vi "lock-in input sweep_1022D.vi"() -> ()   [LabVIEW 2022 SP3]
uses:
  <vilib>/Analysis/baseanly.llb/Mean (DBL).vi
  <vilib>/Utility/file.llb/Write Delimited Spreadsheet (DBL).vi
  <vilib>/Analysis/NI_AALBase.lvlib
panel:
  out "Temperature Status":i32(ring)=1 items=["TemperatureUnknown"=0, "Stable"=1, "Tracking"=2, "Near"=5, "Chasing"=6, "Filling"=7, "Standby"=10, "Disabled"=13, "ImpedanceNotFunction"=14, "TempFailure"=15]
  out "Field Status":i32(ring)=4 items=["MagnetUnknown"=0, "StablePersistent"=1, "WarmingSwitch"=2, "CoolingSwitch"=3, "StableDriven"=4, "Iterating"=5, "Charging"=6, "Discharging"=7, "CurrentError"=8, "MagnetFailure"=15]
  out "Field":dbl=-0.1023246817290783
  out "Temperature":dbl=2.045465922355652
  out "Measuring":bool
  in  "path2 (folder + filename)":string="H:\\My Drive\\Lab\\Opticool\\Measurement\\NLH\\T dependence\\TaI29_A1112_B116"
  in  "Series Resistance":string="20kOhm"
  in  "path1 (folder + filename)":string="H:\\My Drive\\Lab\\Opticool\\Measurement\\NLH\\T dependence\\TaI27_A1016_B1516"
  out "XY Graph 8":cluster{dbl[], dbl[]}(graph)={[0.1], [0.0]}
  out "XY Graph 7":cluster{dbl[], dbl[]}(graph)={[0.1], [0.0]}
  out "XY Graph 6":cluster{dbl[], dbl[]}(graph)
  out "XY Graph 5":cluster{dbl[], dbl[]}(graph)={[0.1], [0.0]}
  out "phase 2B":dbl
  in  "Phase 2B":u16(ring)=9 items=["X", "Y", "R", "Theta", "Frequency", "Noise", "Xh1", "Yh1", "Rh1", "Theta h1", "Xh2", "Yh2", "Rh2", "Theta h2"]
  out "phase 2A":dbl
  in  "Phase 2A":u16(ring)=3 items=["X", "Y", "R", "Theta", "Frequency", "Noise", "Xh1", "Yh1", "Rh1", "Theta h1", "Xh2", "Yh2", "Rh2", "Theta h2"]
  out "para2A Measurement":dbl
  in  "Clear Plot 2A":bool
  in  "Parameter 2A":u16(ring)=2 items=["X", "Y", "R", "Theta", "Frequency", "Noise", "Xh1", "Yh1", "Rh1", "Theta h1", "Xh2", "Yh2", "Rh2", "Theta h2"]
  out "para2B Measurement":dbl
  in  "Clear Plot 2B":bool
  in  "Parameter 2B":u16(ring)=8 items=["X", "Y", "R", "Theta", "Frequency", "Noise", "Xh1", "Yh1", "Rh1", "Theta h1", "Xh2", "Yh2", "Rh2", "Theta h2"]
  in  "Two Lock-in ?":bool=TRUE
  in  "B frequency 2":dbl=267.77 format="%#_13g"
  in  "2B Input Connection (0: Single-Ended)":u16(ring)=1 items=["Single-Ended Voltage", "Differential Voltage", "1 MOhm Current Gain", "100 MOhm Current Gain"]
  in  "2B harmonic 1":u8=2
  in  "2B harmonic 2":u8=3
  in  "2B reference Manual Phase":dbl=-59.75
  in  "auto phase 2B":bool=TRUE
  in  "2B Sample time (s)":dbl=0.001 min=0.001 max=100.0 step=0.001
  in  "2B Sensitivity":u16(ring)=27 items=["1 nV/fA", "2 nV/fA", "5 nV/fA", "10 nV/fA", "20 nV/fA", "50 nV/fA", "100 nV/fA", "200 nV/fA", "500 nV/fA", "1 uV/pA", "2 uV/pA", "5 uV/pA", "10 uV/pA", "20 uV/pA", "50 uV/pA", "100 uV/pA", "200 uV/pA", "500 uV/pA", "1 mV/nA", "2 mV/nA", "5 mV/nA", "10 mV/nA", "20 mV/nA", "50 mV/nA", "100 mV/nA", "200 mV/nA", "500 mV/nA", "1 V/uA"]
  in  "Enable Sync Filter 2B (open when f<200Hz)":bool
  in  "2B Time Constant":u8(ring)=9 items=["10 us", "30 us", "100 us", "300 us", "1 ms", "3 ms", "10 ms", "30 ms", "100 ms", "300 ms", "1 s", "3 s", "10 s", "30 s", "100 s", "300 s", "1 ks", "3 ks"]
  in  "2B Reference Source":u8(ring)=3 items=["External", "Internal", "Internal Sweep", "Channel-A"]
  in  "2B Low Pass Filter Slope":u8(ring)=2 items=["6 dB/oct", "12 dB/oct", "18 db/oct", "24 dB/oct"]
  in  "2A frequency":dbl=267.77 format="%#_13g"
  in  "2A Input Connection (0: Single-Ended)":u16(ring)=1 items=["Single-Ended Voltage", "Differential Voltage", "1 MOhm Current Gain", "100 MOhm Current Gain"]
  in  "2A harmonic":u8=2
  in  "2A harmonic":u8=3
  in  "2A reference Manual Phase":dbl=-59.75
  in  "auto phase 2A":bool=TRUE
  in  "2A Reference Source":u8(ring)=1 items=["External", "Internal", "Internal Sweep"]
  in  "2A Sample time (s)":dbl=0.001 min=0.001 max=100.0 step=0.001
  in  "2A Time Constant":u8(ring)=9 items=["10 us", "30 us", "100 us", "300 us", "1 ms", "3 ms", "10 ms", "30 ms", "100 ms", "300 ms", "1 s", "3 s", "10 s", "30 s", "100 s", "300 s", "1 ks", "3 ks"]
  in  "Enable Sync Filter 2A (open when f<200Hz)":bool
  in  "2A Sensitivity":u16(ring)=27 items=["1 nV/fA", "2 nV/fA", "5 nV/fA", "10 nV/fA", "20 nV/fA", "50 nV/fA", "100 nV/fA", "200 nV/fA", "500 nV/fA", "1 uV/pA", "2 uV/pA", "5 uV/pA", "10 uV/pA", "20 uV/pA", "50 uV/pA", "100 uV/pA", "200 uV/pA", "500 uV/pA", "1 mV/nA", "2 mV/nA", "5 mV/nA", "10 mV/nA", "20 mV/nA", "50 mV/nA", "100 mV/nA", "200 mV/nA", "500 mV/nA", "1 V/uA"]
  in  "2A Low Pass Filter Slope":u8(ring)=2 items=["6 dB/oct", "12 dB/oct", "18 db/oct", "24 dB/oct"]
  in  "LOCKIN2 address":refnum<visa-resource-name>="COM3"
  in  "Temperature \n& Field Function":bool
  in  "Field Approach":i32(ring) items=["Linear", "NoOvershoot", "Oscillate"]
  in  "F Rate (Oe/s)":dbl=100.0 format="%#_13g"
  in  "Set F (Oe)":dbl format="%#_13g"
  in  "Mode":i32(ring) items=["Persistent", "Driven"]
  in  "Temperature Approach":i32(ring)=1 items=["FastSettle", "NoOvershoot"]
  in  "T  Rate (K/min)":dbl=10.0
  in  "Set  T  (K)":dbl=2.0
  in  "WaitForField":bool=TRUE
  in  "WaitForTemperature":bool=TRUE
  in  "Delay":dbl=5.0
  in  "Remote":bool=TRUE
  in  "IP Address":string="169.254.170.239"
  in  "1A Low Pass Filter Slope":u8(ring)=2 items=["6 dB/oct", "12 dB/oct", "18 db/oct", "24 dB/oct"]
  in  "1B Low Pass Filter Slope":u8(ring)=2 items=["6 dB/oct", "12 dB/oct", "18 db/oct", "24 dB/oct"]
  in  "1B Reference Source":u8(ring)=3 items=["External", "Internal", "Internal Sweep", "Channel-A"]
  in  "1B Time Constant":u8(ring)=9 items=["10 us", "30 us", "100 us", "300 us", "1 ms", "3 ms", "10 ms", "30 ms", "100 ms", "300 ms", "1 s", "3 s", "10 s", "30 s", "100 s", "300 s", "1 ks", "3 ks"]
  in  "Enable Sync Filter 1B (open f<200Hz)":bool
  in  "1B Sensitivity":u16(ring)=27 items=["1 nV/fA", "2 nV/fA", "5 nV/fA", "10 nV/fA", "20 nV/fA", "50 nV/fA", "100 nV/fA", "200 nV/fA", "500 nV/fA", "1 uV/pA", "2 uV/pA", "5 uV/pA", "10 uV/pA", "20 uV/pA", "50 uV/pA", "100 uV/pA", "200 uV/pA", "500 uV/pA", "1 mV/nA", "2 mV/nA", "5 mV/nA", "10 mV/nA", "20 mV/nA", "50 mV/nA", "100 mV/nA", "200 mV/nA", "500 mV/nA", "1 V/uA"]
  in  "1A Sensitivity":u16(ring)=27 items=["1 nV/fA", "2 nV/fA", "5 nV/fA", "10 nV/fA", "20 nV/fA", "50 nV/fA", "100 nV/fA", "200 nV/fA", "500 nV/fA", "1 uV/pA", "2 uV/pA", "5 uV/pA", "10 uV/pA", "20 uV/pA", "50 uV/pA", "100 uV/pA", "200 uV/pA", "500 uV/pA", "1 mV/nA", "2 mV/nA", "5 mV/nA", "10 mV/nA", "20 mV/nA", "50 mV/nA", "100 mV/nA", "200 mV/nA", "500 mV/nA", "1 V/uA"]
  in  "Enable Sync Filter 1A (open f<200Hz)":bool
  in  "1A Time Constant":u8(ring)=9 items=["10 us", "30 us", "100 us", "300 us", "1 ms", "3 ms", "10 ms", "30 ms", "100 ms", "300 ms", "1 s", "3 s", "10 s", "30 s", "100 s", "300 s", "1 ks", "3 ks"]
  out "XY Graph 4":cluster{dbl[], dbl[]}(graph)={[0.1], [18.0]}
  in  "Phase 1B":u16(ring)=9 items=["X", "Y", "R", "Theta", "Frequency", "Noise", "Xh1", "Yh1", "Rh1", "Theta h1", "Xh2", "Yh2", "Rh2", "Theta h2"]
  in  "Parameter 1B":u16(ring)=8 items=["X", "Y", "R", "Theta", "Frequency", "Noise", "Xh1", "Yh1", "Rh1", "Theta h1", "Xh2", "Yh2", "Rh2", "Theta h2"]
  out "phase 1B":dbl=18.0
  in  "Clear Plot 1B":bool
  out "XY Graph 3":cluster{dbl[], dbl[]}(graph)={[0.1], [0.0]}
  out "para1B Measurement":dbl
  out "XY Graph 2":cluster{dbl[], dbl[]}(graph)={[0.1], [18.672111582001435]}
  in  "1B Sample time (s)":dbl=0.001 min=0.001 max=100.0 step=0.001
  in  "1A Sample time (s)":dbl=0.001 min=0.001 max=100.0 step=0.001
  in  "Phase 1A":u16(ring)=3 items=["X", "Y", "R", "Theta", "Frequency", "Noise", "Xh1", "Yh1", "Rh1", "Theta h1", "Xh2", "Yh2", "Rh2", "Theta h2"]
  in  "Parameter 1A":u16(ring)=2 items=["X", "Y", "R", "Theta", "Frequency", "Noise", "Xh1", "Yh1", "Rh1", "Theta h1", "Xh2", "Yh2", "Rh2", "Theta h2"]
  in  "stabilization(S)":dbl=0.5 format="%#_13g"
  in  "1B frequency":dbl=267.77 format="%#_13g"
  in  "1B Input Connection (0: Single-Ended)":u16(ring)=1 items=["Single-Ended Voltage", "Differential Voltage", "1 MOhm Current Gain", "100 MOhm Current Gain"]
  in  "1B harmonic 1":u8=2
  in  "B harmonic 2":u8=3
  in  "1B reference Manual Phase":dbl=-59.75
  in  "auto phase 1B":bool=TRUE
  in  "1A frequency":dbl=267.77 format="%#_13g"
  in  "1A Input Connection (0: Single-Ended)":u16(ring)=1 items=["Single-Ended Voltage", "Differential Voltage", "1 MOhm Current Gain", "100 MOhm Current Gain"]
  in  "1A harmonic 1":u8=2
  in  "1A harmonic 2":u8=3
  in  "1A reference Manual Phase":dbl=-59.75
  in  "auto phase 1A":bool=TRUE
  in  "1A Reference Source":u8(ring)=1 items=["External", "Internal", "Internal Sweep"]
  out "phase 1A":dbl=18.672111582001435
  out "loop run":i32=1
  in  "loop #":i32=1
  in  "Save data or not":bool=TRUE
  in  "Clear Plot 1A":bool
  out "XY Graph":cluster{dbl[], dbl[]}(graph)={[0.1], [2.9721208903815985]}
  out "para1A Measurement":dbl=2.9721208903815985
  out "Sine voltage":dbl=0.1 format="%#_13g"
  in  "GATE STEP(mv)":i32=20
  in  "Sine Low Value (0V)":dbl=0.1
  in  "Sine High Value (0.001-5V)":dbl=3.0
  in  "lockin waiting (s)":dbl=0.1 format="%#_13g"
  in  "LOCKIN1 address":refnum<visa-resource-name>="COM4"
  # "Mesurement 1"
  # "Lock-in 1 Setting"
  # "Channel 1A"
  # "Channel 1B"
  # "Lock-in 2 Setting"
  # "Channel 2A"
  # "Channel 2B"
  # "Mesurement 2"
  # "Mesurement 1"
  # "Sine Sweep Setting (Channel 1A)"
  # "Temprature and Field Setting"
  # "Mesurement 2"
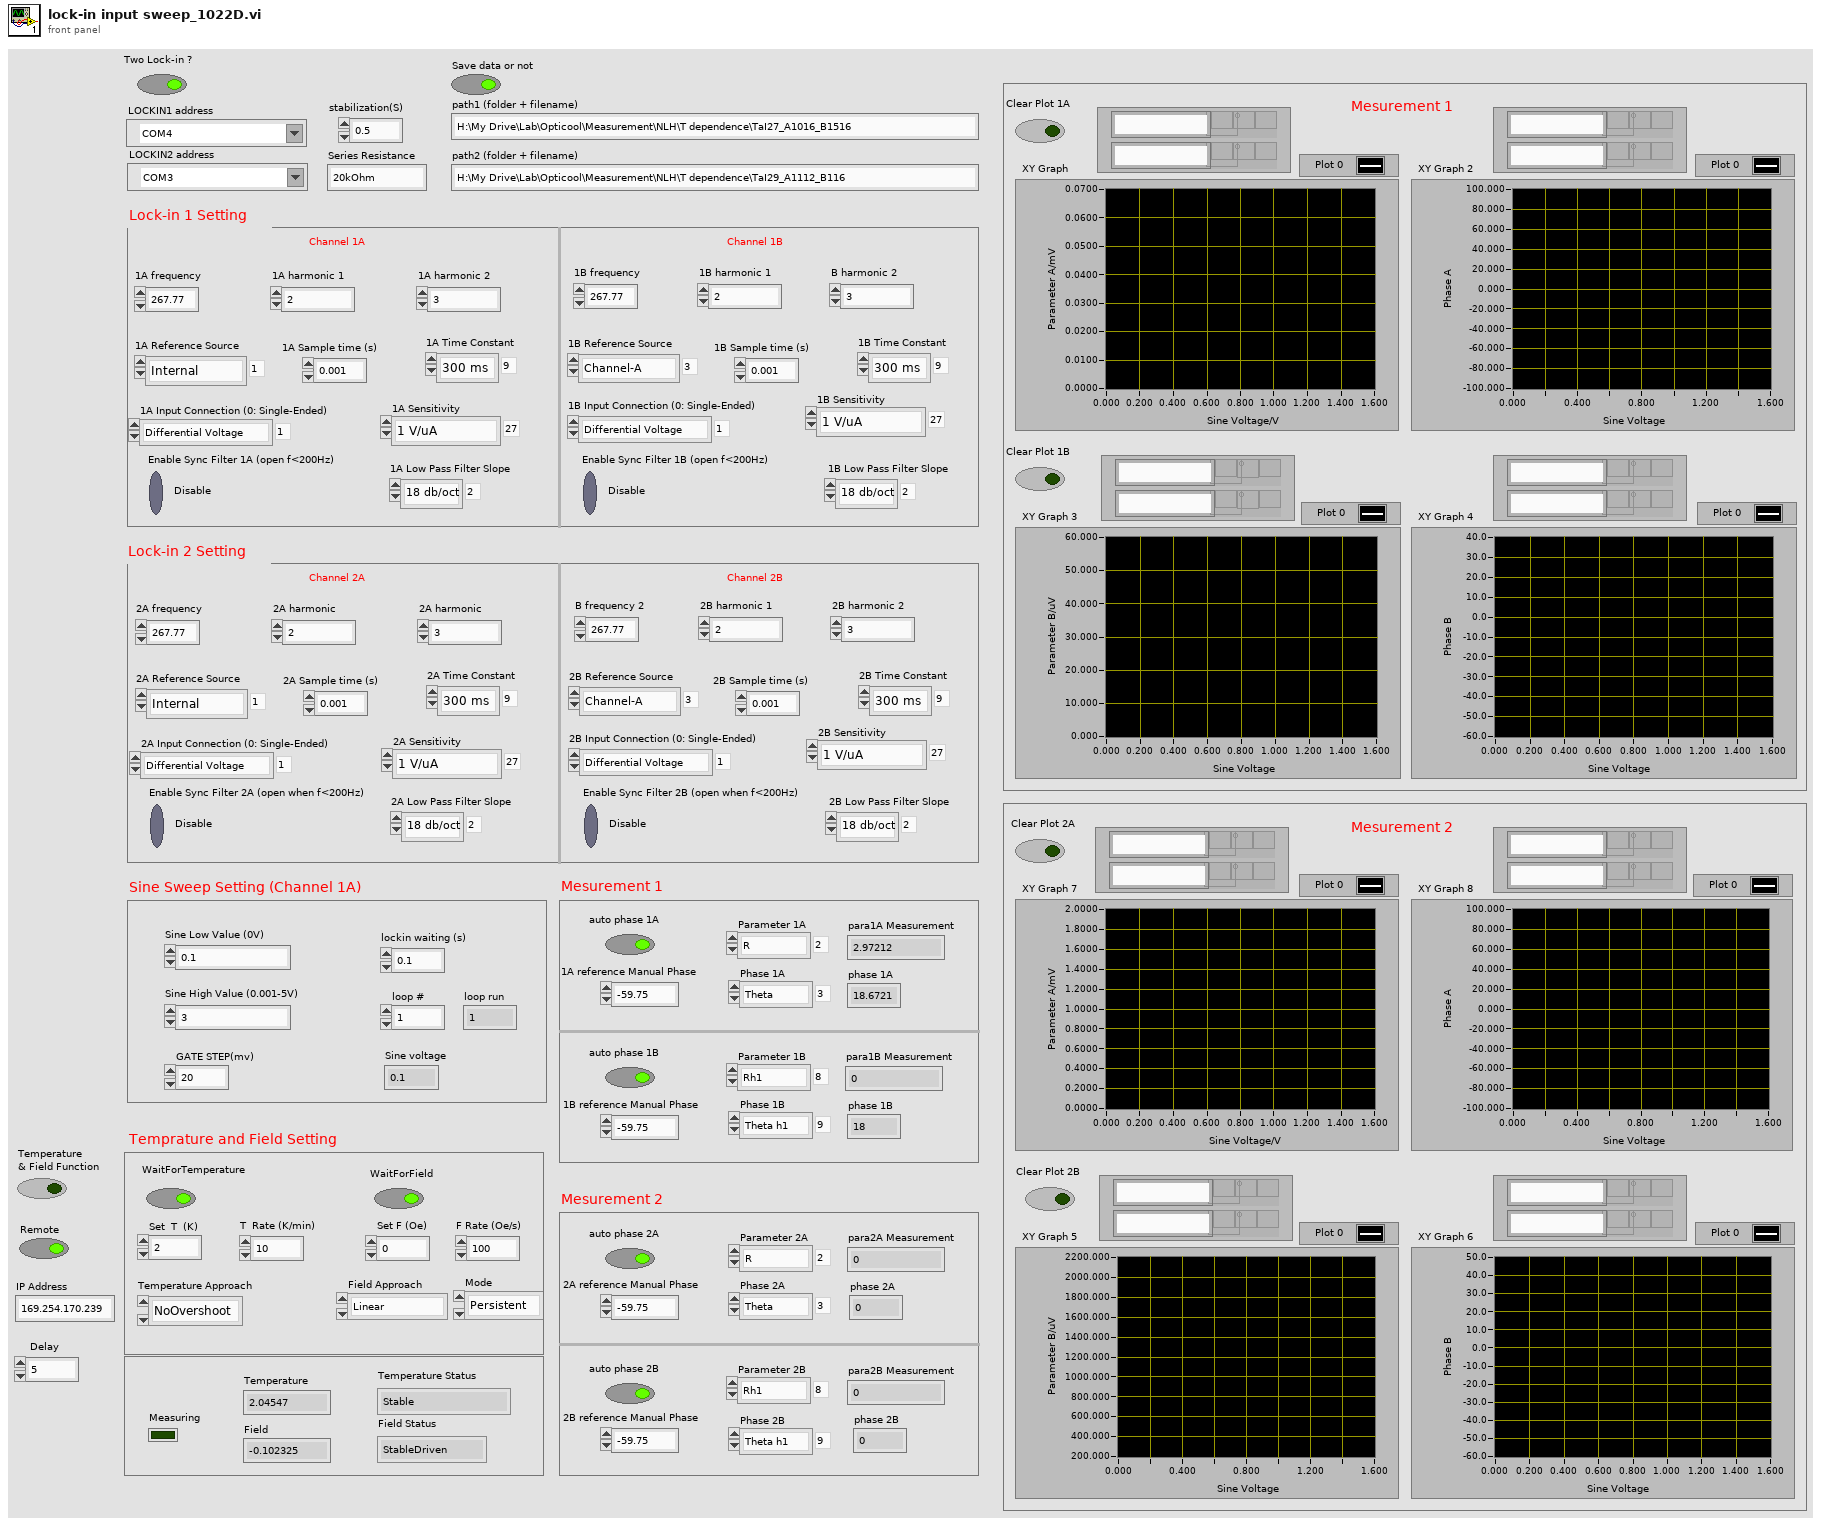
[diagram p1: front panel]
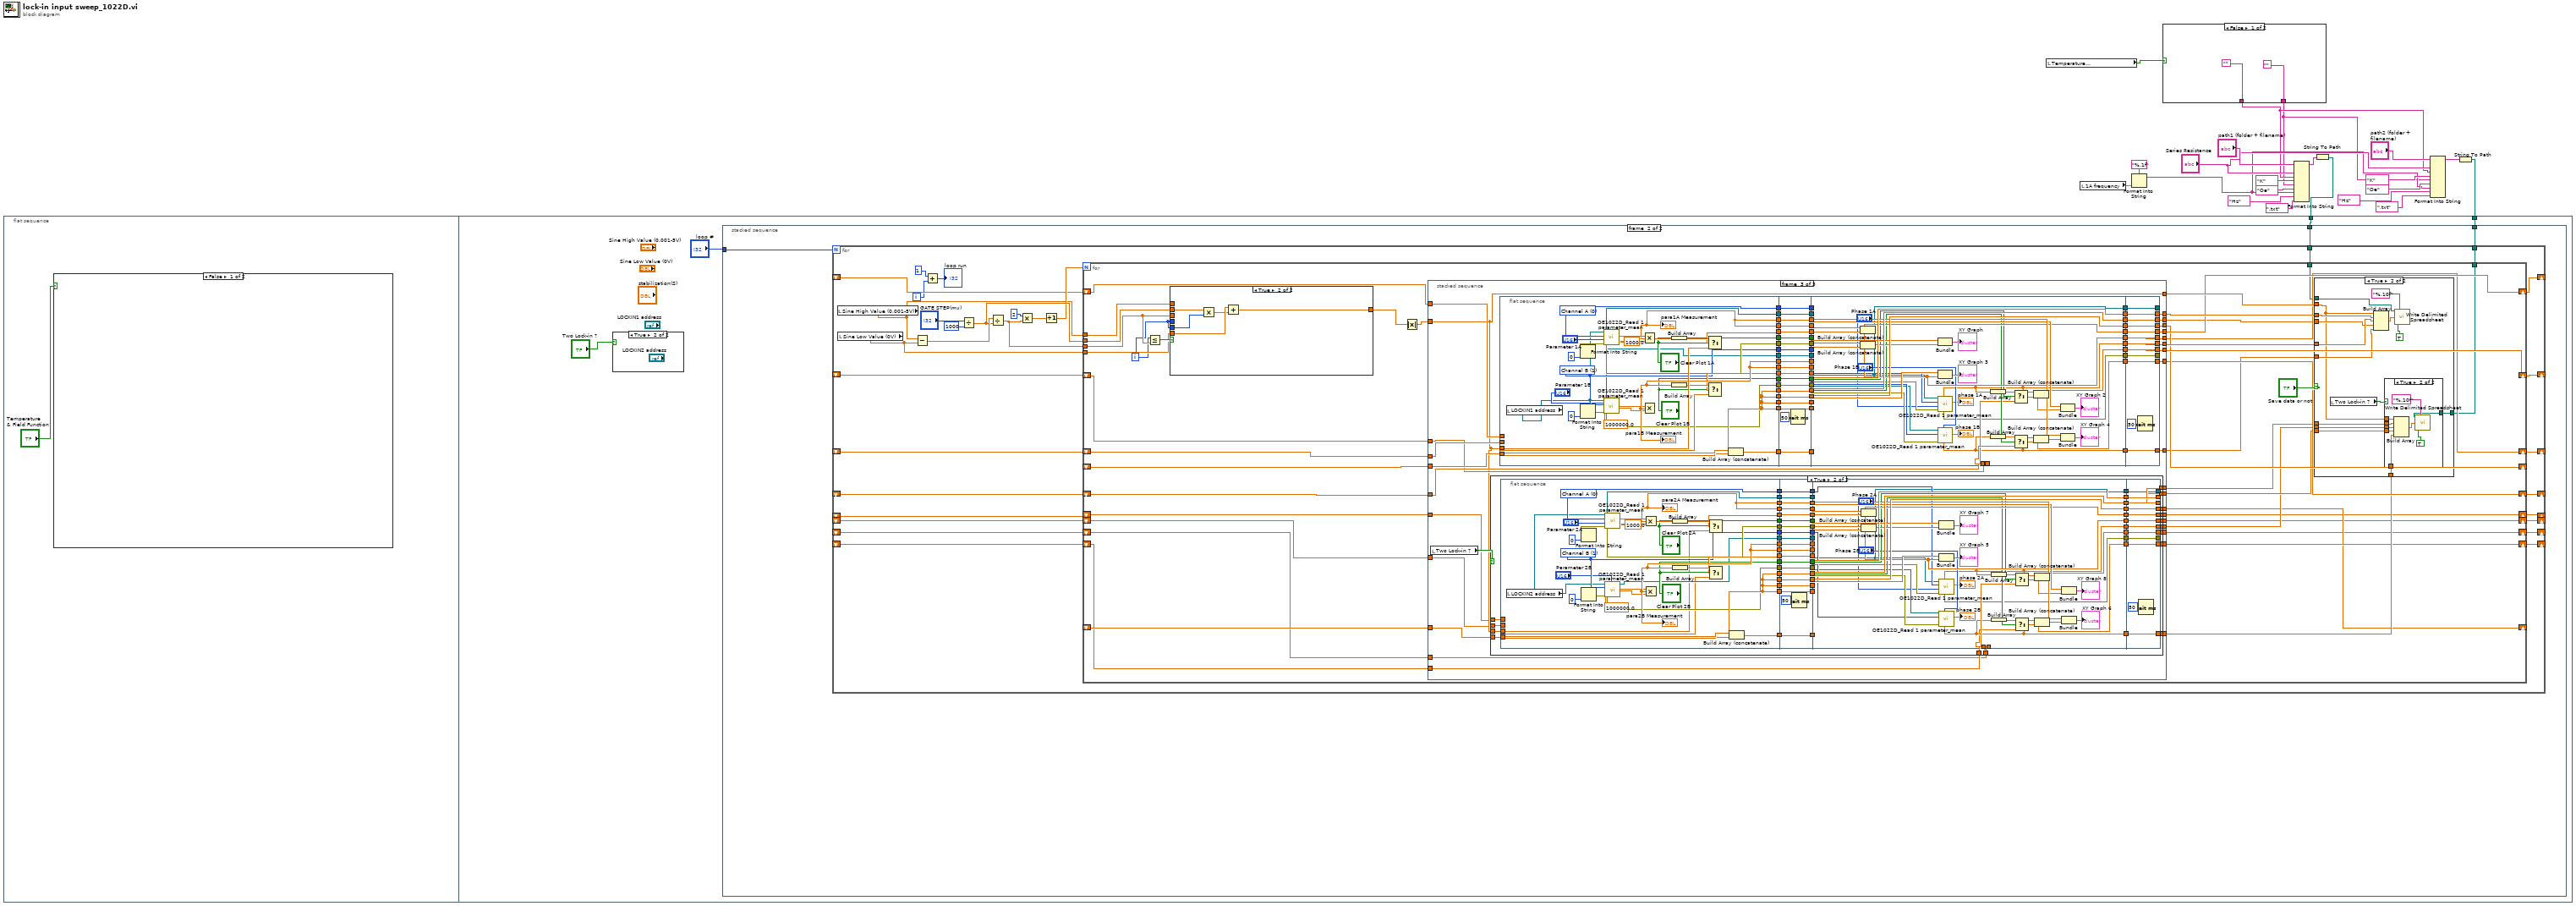
[diagram p0: block diagram]
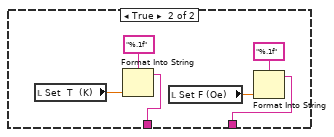
[diagram p2: hidden frame]
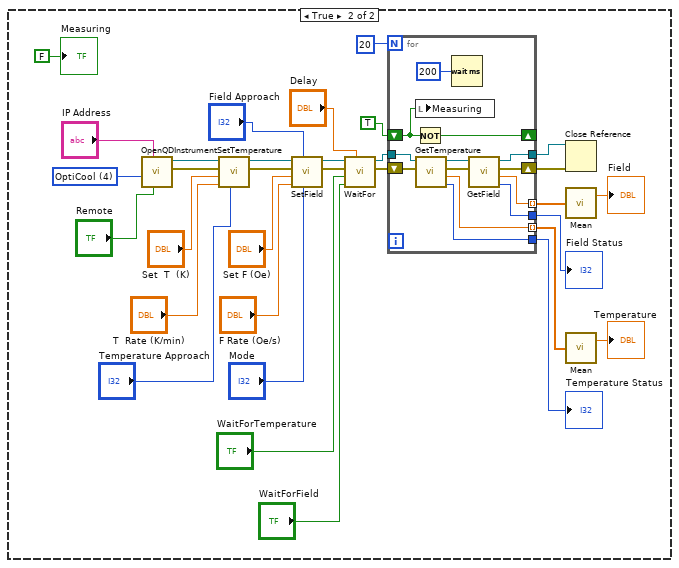
[diagram p3: hidden frame]
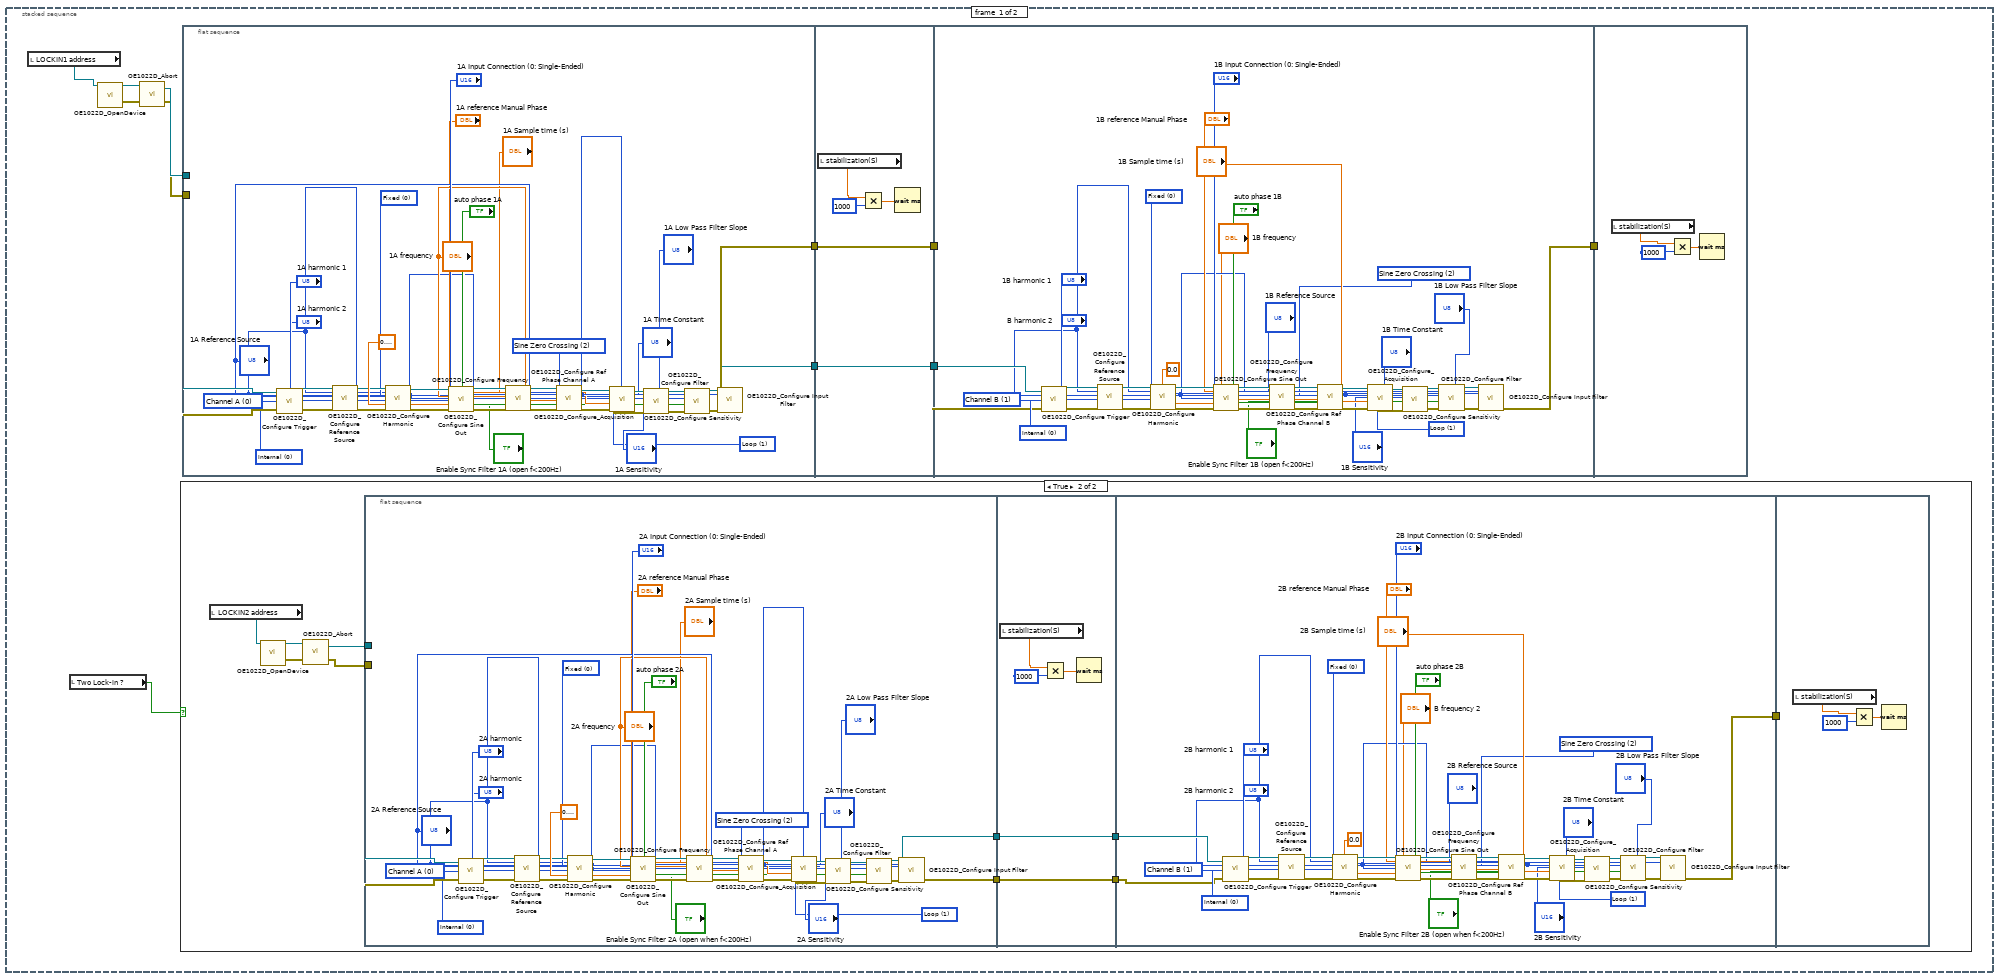
[diagram p5: hidden frame]
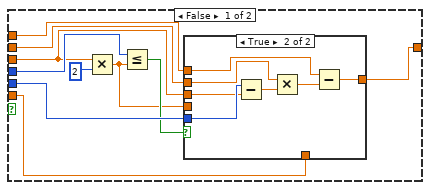
[diagram p9: hidden frame]
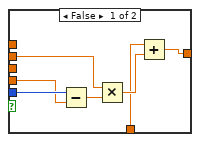
[diagram p10: hidden frame]
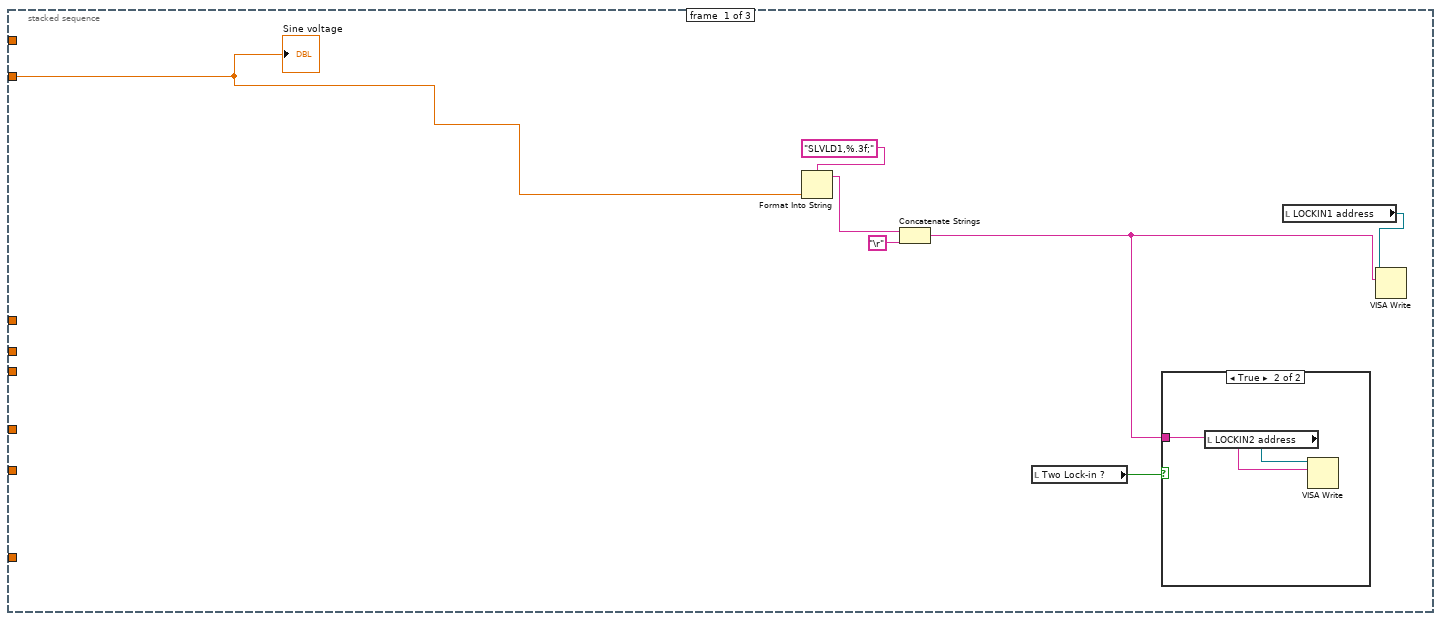
[diagram p11: hidden frame]
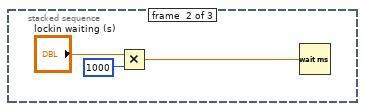
[diagram p13: hidden frame]
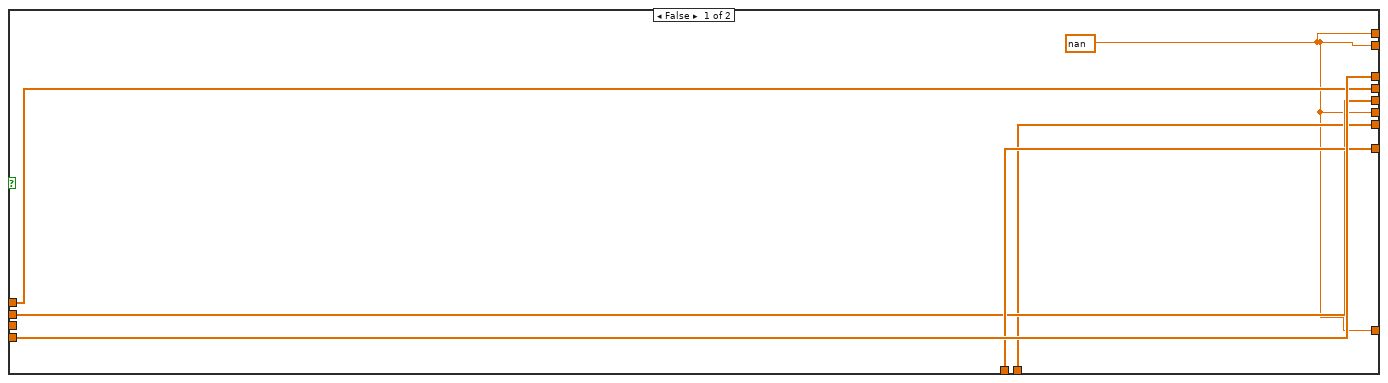
[diagram p14: hidden frame]
diagram:
  n1 = flat-sequence {
    tunnel: w16 -> [w69]
    tunnel: w1 -> [w68]
    frame #0 {
      n2 = case shown="False" "Temperature \n& Field Function" {
        frame False {
        }
        frame True {
          w46 = 4 items=["PPMS", "VersaLab", "DynaCool", "SVSM", "OptiCool"] ("InstrumentType")
          n3 = call "OpenQDInstrument.vi"("Remote"="Remote", "IP Address"="IP Address", "InstrumentType"=w46) -> ("error out"=w37:errorcluster, "Instrument Ref"=w38:refnum<k24>)  [unwired: 5 in]
          n4 = call "SetTemperature.vi"("Approach"="Temperature Approach", "Rate"="T  Rate (K/min)", "Temperature"="Set  T  (K)", "error in (no error)"=w37, "Instrument Ref In"=w38) -> ("error out"=w51:errorcluster, "Instrument Ref Out"=w50:refnum<k24>)  [unwired: 2 in, 1 out]
          n5 = call "SetField.vi"("Mode"="Mode", "Approach"="Field Approach", "Rate"="F Rate (Oe/s)", "Field"="Set F (Oe)", "error in (no error)"=w51, "Instrument Ref In"=w50) -> ("error out"=w33:errorcluster, "Instrument Ref Out"=w34:refnum<k24>)  [unwired: 1 in, 1 out]
          n6 = call "WaitFor.vi"("Delay"="Delay", "Wait For Field"="WaitForField", "Wait For Temperature"="WaitForTemperature", "error in (no error)"=w33, "Instrument Ref In"=w34) -> ("error out"=w45:errorcluster, "Instrument Ref Out"=w41:refnum<k24>)  [unwired: 5 in]
          n7 = for {
            N: 20 -> [_]
            shift-right: [w67] -> _
            shift-left: TRUE -> [w65]
            shift-right: [w62] -> w35
            shift-left: w45 -> [w64]
            tunnel: w41 -> [w61]
            tunnel: [w59] -> w36
            tunnel: [w56] -> w24
            tunnel: [w55] -> w23
            tunnel: [w57] -> w39 mode=indexing
            tunnel: [w58] -> w40 mode=indexing
            n8 = Not(x=w65) -> (.not. x?=w67:bool)
            n9 = local write "Measuring"(w65) -> ()
            n10 = call "GetTemperature.vi"("error in (no error)"=w64, "Instrument Ref In"=w61) -> ("Temperature\nStatus"=w55:i32, "Temperature"=w58:dbl, "error out"=w63:errorcluster, "Instrument Ref Out"=w60:refnum<k24>)  [unwired: 3 in, 1 out]
            n11 = Wait (ms)(milliseconds to wait=u32 200) -> ()  [unwired: 1 out]
            n12 = call "GetField.vi"("error in (no error)"=w63, "Instrument Ref In"=w60) -> ("Field\nStatus"=w56:i32, "Field"=w57:dbl, "error out"=w62:errorcluster, "Instrument Ref Out"=w59:refnum<k24>)  [unwired: 3 in, 1 out]
          }
          "Field Status" <- w24
          "Temperature Status" <- w23
          n13 = Close Reference(reference=w36, error in (no error)=w35) -> ()  [unwired: 1 out]
          n14 = call-poly <vilib>:"Mean.vi"("X"=w39) -> ("mean"=→"Field":dbl)  [unwired: 1 out]
          n15 = call-poly <vilib>:"Mean.vi"("X"=w40) -> ("mean"=→"Temperature":dbl)  [unwired: 1 out]
          "Measuring" <- FALSE
        }
      }
    }
    frame #1 {
      n16 = case shown="True" "Two Lock-in ?" {
        frame False {
        }
        frame True {
        }
      }
      n17 = stacked-sequence {
        tunnel: "loop #" -> [_ w269]
        tunnel: w69 -> [_ w268]
        tunnel: w68 -> [_ w267]
        frame #0 {
          n18 = local read "LOCKIN1 address"() -> (w73:refnum<visa-resource-name>)
          n19 = local read "Two Lock-in ?"() -> (w72:bool)
          n20 = call "OE1022D_OpenDevice.vi"("VISA resource name"=w73) -> ("VISA资源名称输出"=w74:refnum<visa-resource-name>, "错误输出"=w75:errorcluster)  [unwired: 17 in]
          n21 = call "OE1022D_Abort.vi"("error in (no error)"=w75, "VISA resource name"=w74) -> ("error out"=w80:errorcluster, "VISA resource name out"=w81:refnum<visa-resource-name>)
          n22 = case shown="True" w72 {
            frame False {
            }
            frame True {
              n23 = local read "LOCKIN2 address"() -> (w83:refnum<visa-resource-name>)
              n24 = call "OE1022D_OpenDevice.vi"("VISA resource name"=w83) -> ("VISA资源名称输出"=w86:refnum<visa-resource-name>, "错误输出"=w87:errorcluster)  [unwired: 17 in]
              n25 = call "OE1022D_Abort.vi"("error in (no error)"=w87, "VISA resource name"=w86) -> ("error out"=w84:errorcluster, "VISA resource name out"=w85:refnum<visa-resource-name>)
              n26 = flat-sequence {
                tunnel: w85 -> [w132]
                tunnel: [w120] -> w92
                tunnel: w84 -> [w131]
                tunnel: [w108] -> w91
                tunnel: w92 -> [w137]
                tunnel: [w137] -> w90
                tunnel: w91 -> [w136]
                tunnel: [w136] -> w89
                tunnel: w90 -> [w159]
                tunnel: [w158] -> w88
                tunnel: w89 -> [w157]
                tunnel: w88 -> [_]
                frame #0 {
                  w93 = u8 2 items=["TTL Pos", "TTL Neg", "Sine Zero Crossing"] ("External Ref Trigger")
                  w94 = u8 1 items=["Single", "Loop"] ("Sample Mode (Single/Loop)")
                  w107 = u8 0 items=["Fixed", "Linear", "Log"] ("SineOut Mode")
                  w109 = u16 0 items=["Internal", "External"] ("Trigger Source (0: Internal)")
                  w98 = u8 0 items=["Channel A", "Channel B"] ("OE1022D A/B")
                  n27 = call "OE1022D_Configure Trigger.vi"("Trigger Source (0: Internal)"=w109, "error in (no error)   2"=w131, "OE1022D A/B"=w98, "VISA resource name   2"=w132) -> ("error out   2"=w125:errorcluster, "VISA resource name out   2"=w126:refnum<visa-resource-name>)
                  n28 = call "OE1022D_Configure Reference Source.vi"("VISA resource name"=w126, "OE1022D A/B"=w98, "Reference Source"="2A Reference Source", "error in (no error)"=w125) -> ("VISA resource name out"=w124:refnum<visa-resource-name>, "error out"=w122:errorcluster)  [unwired: 14 in]
                  n29 = call "OE1022D_Configure Harmonic.vi"("VISA resource name"=w124, "OE1022D A/B"=w98, "Harmonic 1"="2A harmonic", "Harmonic 2"="2A harmonic", "error in (no error)"=w122) -> ("VISA resource name out"=w123:refnum<visa-resource-name>, "error out"=w121:errorcluster)  [unwired: 13 in]
                  n30 = call "OE1022D_Configure Sine Out.vi"("VISA resource name"=w123, "SineOut Mode"=w107, "OE1022D A/B"=w98, "Sine Output Amplitude (V)"=sgl 0.1, "error in (no error)"=w121) -> ("VISA resource name out"=w129:refnum<visa-resource-name>, "error out"=w128:errorcluster)  [unwired: 9 in]
                  n31 = call "OE1022D_Configure Frequency.vi"("VISA resource name"=w129, "OE1022D A/B"=w98, "Internal Frequency(Hz)"="2A frequency", "error in (no error)"=w128) -> ("VISA resource name out"=w119:refnum<visa-resource-name>, "error out"=w116:errorcluster)  [unwired: 14 in]
                  n32 = call "OE1022D_Configure Ref Phase Channel A.vi"("VISA resource name"=w119, "Reference Source"="2A Reference Source", "External Ref Trigger"=w93, "Internal Frequency(Hz)"="2A frequency", "Auto Phase (T: Enabled)"="auto phase 2A", "error in (no error)"=w116, "Manual Phase  (degree)"="2A reference Manual Phase") -> ("VISA resource name out"=w118:refnum<visa-resource-name>, "error out"=w117:errorcluster)  [unwired: 11 in]
                  n33 = call "OE1022D_Configure_Acquisition.vi"("VISA resource name"=w118, "OE1022D A/B"=w98, "Sample time (s)"="2A Sample time (s)", "error in (no error)"=w117, "Sample Mode (Single/Loop)"=w94) -> ("VISA resource name out"=w101:refnum<visa-resource-name>, "error out"=w100:errorcluster)  [unwired: 3 in]
                  n34 = call "OE1022D_Configure Sensitivity.vi"("VISA resource name"=w101, "OE1022D A/B"=w98, "Sensitivity"="2A Sensitivity", "error in (no error)"=w100) -> ("VISA resource name out"=w105:refnum<visa-resource-name>, "error out"=w104:errorcluster)  [unwired: 14 in]
                  n35 = call "OE1022D_Configure Filter.vi"("Low Pass Filter Slope (1: 12dB/oct)"="2A Low Pass Filter Slope", "Time Constant (8: 100ms)"="2A Time Constant", "error in (no error)"=w104, "Enable Sync Filter (F: Disable)"="Enable Sync Filter 2A (open when f<200Hz)", "OE1022D A/B"=w98, "VISA resource name"=w105) -> ("error out"=w102:errorcluster, "VISA resource name out"=w103:refnum<visa-resource-name>)  [unwired: 4 in]
                  n36 = call "OE1022D_Configure Input Filter.vi"("VISA resource name"=w103, "Input Source"="2A Input Connection (0: Single-Ended)", "OE1022D A/B"=w98, "error in (no error)"=w102) -> ("VISA resource name out"=w108:refnum<visa-resource-name>, "error out"=w120:errorcluster)  [unwired: 10 in]
                }
                frame #1 {
                  n37 = local read "stabilization(S)"() -> (w133:dbl)
                  n38 = Multiply(x=w133, y=1000) -> (x*y=w135:dbl)
                  n39 = Wait (ms)(milliseconds to wait=w135) -> ()  [unwired: 1 out]
                }
                frame #2 {
                  w139 = u8 1 items=["Single", "Loop"] ("Sample Mode (Single/Loop)")
                  w141 = u8 2 items=["TTL Pos", "TTL Neg", "Sine Zero Crossing"] ("External Ref Trigger")
                  w154 = u8 0 items=["Fixed", "Linear", "Log"] ("SineOut Mode")
                  w160 = u16 0 items=["Internal", "External"] ("Trigger Source (0: Internal)")
                  w146 = u8 1 items=["Channel A", "Channel B"] ("OE1022D A/B")
                  n40 = call "OE1022D_Configure Trigger.vi"("Trigger Source (0: Internal)"=w160, "error in (no error)   2"=w159, "OE1022D A/B"=w146, "VISA resource name   2"=w157) -> ("error out   2"=w172:errorcluster, "VISA resource name out   2"=w173:refnum<visa-resource-name>)
                  n41 = call "OE1022D_Configure Reference Source.vi"("VISA resource name"=w173, "OE1022D A/B"=w146, "error in (no error)"=w172) -> ("VISA resource name out"=w171:refnum<visa-resource-name>, "error out"=w169:errorcluster)  [unwired: 15 in]
                  n42 = call "OE1022D_Configure Harmonic.vi"("VISA resource name"=w171, "OE1022D A/B"=w146, "Harmonic 1"="2B harmonic 1", "Harmonic 2"="2B harmonic 2", "error in (no error)"=w169) -> ("VISA resource name out"=w170:refnum<visa-resource-name>, "error out"=w168:errorcluster)  [unwired: 13 in]
                  n43 = call "OE1022D_Configure Sine Out.vi"("VISA resource name"=w170, "SineOut Mode"=w154, "OE1022D A/B"=w146, "Sine Output Amplitude (V)"=sgl 0.0, "error in (no error)"=w168) -> ("VISA resource name out"=w175:refnum<visa-resource-name>, "error out"=w174:errorcluster)  [unwired: 9 in]
                  n44 = call "OE1022D_Configure Frequency.vi"("VISA resource name"=w175, "OE1022D A/B"=w146, "Internal Frequency(Hz)"="B frequency 2", "error in (no error)"=w174) -> ("VISA resource name out"=w167:refnum<visa-resource-name>, "error out"=w164:errorcluster)  [unwired: 14 in]
                  n45 = call "OE1022D_Configure Ref Phase Channel B.vi"("VISA resource name"=w167, "Reference Source"="2B Reference Source", "External Ref Trigger"=w141, "Internal Frequency(Hz)"="B frequency 2", "Auto Phase (T: Enabled)"="auto phase 2B", "error in (no error)"=w164, "Manual Phase  (degree)"="2B reference Manual Phase") -> ("VISA resource name out"=w166:refnum<visa-resource-name>, "error out"=w165:errorcluster)  [unwired: 11 in]
                  n46 = call "OE1022D_Configure_Acquisition.vi"("VISA resource name"=w166, "OE1022D A/B"=w146, "Sample time (s)"="2B Sample time (s)", "error in (no error)"=w165, "Sample Mode (Single/Loop)"=w139) -> ("VISA resource name out"=w147:refnum<visa-resource-name>, "error out"=w148:errorcluster)  [unwired: 3 in]
                  n47 = call "OE1022D_Configure Sensitivity.vi"("VISA resource name"=w147, "OE1022D A/B"=w146, "Sensitivity"="2B Sensitivity", "error in (no error)"=w148) -> ("VISA resource name out"=w151:refnum<visa-resource-name>, "error out"=w150:errorcluster)  [unwired: 14 in]
                  n48 = call "OE1022D_Configure Filter.vi"("Low Pass Filter Slope (1: 12dB/oct)"="2B Low Pass Filter Slope", "Time Constant (8: 100ms)"="2B Time Constant", "error in (no error)"=w150, "Enable Sync Filter (F: Disable)"="Enable Sync Filter 2B (open when f<200Hz)", "OE1022D A/B"=w146, "VISA resource name"=w151) -> ("error out"=w149:errorcluster, "VISA resource name out"=w138:refnum<visa-resource-name>)  [unwired: 4 in]
                  n49 = call "OE1022D_Configure Input Filter.vi"("VISA resource name"=w138, "Input Source"="2B Input Connection (0: Single-Ended)", "OE1022D A/B"=w146, "error in (no error)"=w149) -> ("error out"=w158:errorcluster)  [unwired: 10 in, 1 out]
                }
                frame #3 {
                  n50 = local read "stabilization(S)"() -> (w177:dbl)
                  n51 = Multiply(x=w177, y=1000) -> (x*y=w179:dbl)
                  n52 = Wait (ms)(milliseconds to wait=w179) -> ()  [unwired: 1 out]
                }
              }
            }
          }
          n53 = flat-sequence {
            tunnel: w81 -> [w219]
            tunnel: [w207] -> w79
            tunnel: w80 -> [w218]
            tunnel: [w195] -> w77
            tunnel: w79 -> [w224]
            tunnel: [w224] -> w78
            tunnel: w77 -> [w223]
            tunnel: [w223] -> w76
            tunnel: w78 -> [w246]
            tunnel: [w245] -> w82
            tunnel: w76 -> [w244]
            tunnel: w82 -> [_]
            frame #0 {
              w180 = u8 2 items=["TTL Pos", "TTL Neg", "Sine Zero Crossing"] ("External Ref Trigger")
              w181 = u8 1 items=["Single", "Loop"] ("Sample Mode (Single/Loop)")
              w194 = u8 0 items=["Fixed", "Linear", "Log"] ("SineOut Mode")
              w196 = u16 0 items=["Internal", "External"] ("Trigger Source (0: Internal)")
              w185 = u8 0 items=["Channel A", "Channel B"] ("OE1022D A/B")
              n54 = call "OE1022D_Configure Trigger.vi"("Trigger Source (0: Internal)"=w196, "error in (no error)   2"=w218, "OE1022D A/B"=w185, "VISA resource name   2"=w219) -> ("error out   2"=w212:errorcluster, "VISA resource name out   2"=w213:refnum<visa-resource-name>)
              n55 = call "OE1022D_Configure Reference Source.vi"("VISA resource name"=w213, "OE1022D A/B"=w185, "Reference Source"="1A Reference Source", "error in (no error)"=w212) -> ("VISA resource name out"=w211:refnum<visa-resource-name>, "error out"=w209:errorcluster)  [unwired: 14 in]
              n56 = call "OE1022D_Configure Harmonic.vi"("VISA resource name"=w211, "OE1022D A/B"=w185, "Harmonic 1"="1A harmonic 1", "Harmonic 2"="1A harmonic 2", "error in (no error)"=w209) -> ("VISA resource name out"=w210:refnum<visa-resource-name>, "error out"=w208:errorcluster)  [unwired: 13 in]
              n57 = call "OE1022D_Configure Sine Out.vi"("VISA resource name"=w210, "SineOut Mode"=w194, "OE1022D A/B"=w185, "Sine Output Amplitude (V)"=sgl 0.1, "error in (no error)"=w208) -> ("VISA resource name out"=w216:refnum<visa-resource-name>, "error out"=w215:errorcluster)  [unwired: 9 in]
              n58 = call "OE1022D_Configure Frequency.vi"("VISA resource name"=w216, "OE1022D A/B"=w185, "Internal Frequency(Hz)"="1A frequency", "error in (no error)"=w215) -> ("VISA resource name out"=w206:refnum<visa-resource-name>, "error out"=w203:errorcluster)  [unwired: 14 in]
              n59 = call "OE1022D_Configure Ref Phase Channel A.vi"("VISA resource name"=w206, "Reference Source"="1A Reference Source", "External Ref Trigger"=w180, "Internal Frequency(Hz)"="1A frequency", "Auto Phase (T: Enabled)"="auto phase 1A", "error in (no error)"=w203, "Manual Phase  (degree)"="1A reference Manual Phase") -> ("VISA resource name out"=w205:refnum<visa-resource-name>, "error out"=w204:errorcluster)  [unwired: 11 in]
              n60 = call "OE1022D_Configure_Acquisition.vi"("VISA resource name"=w205, "OE1022D A/B"=w185, "Sample time (s)"="1A Sample time (s)", "error in (no error)"=w204, "Sample Mode (Single/Loop)"=w181) -> ("VISA resource name out"=w188:refnum<visa-resource-name>, "error out"=w187:errorcluster)  [unwired: 3 in]
              n61 = call "OE1022D_Configure Sensitivity.vi"("VISA resource name"=w188, "OE1022D A/B"=w185, "Sensitivity"="1A Sensitivity", "error in (no error)"=w187) -> ("VISA resource name out"=w192:refnum<visa-resource-name>, "error out"=w191:errorcluster)  [unwired: 14 in]
              n62 = call "OE1022D_Configure Filter.vi"("Low Pass Filter Slope (1: 12dB/oct)"="1A Low Pass Filter Slope", "Time Constant (8: 100ms)"="1A Time Constant", "error in (no error)"=w191, "Enable Sync Filter (F: Disable)"="Enable Sync Filter 1A (open f<200Hz)", "OE1022D A/B"=w185, "VISA resource name"=w192) -> ("error out"=w189:errorcluster, "VISA resource name out"=w190:refnum<visa-resource-name>)  [unwired: 4 in]
              n63 = call "OE1022D_Configure Input Filter.vi"("VISA resource name"=w190, "Input Source"="1A Input Connection (0: Single-Ended)", "OE1022D A/B"=w185, "error in (no error)"=w189) -> ("VISA resource name out"=w195:refnum<visa-resource-name>, "error out"=w207:errorcluster)  [unwired: 10 in]
            }
            frame #1 {
              n64 = local read "stabilization(S)"() -> (w220:dbl)
              n65 = Multiply(x=w220, y=1000) -> (x*y=w222:dbl)
              n66 = Wait (ms)(milliseconds to wait=w222) -> ()  [unwired: 1 out]
            }
            frame #2 {
              w226 = u8 1 items=["Single", "Loop"] ("Sample Mode (Single/Loop)")
              w228 = u8 2 items=["TTL Pos", "TTL Neg", "Sine Zero Crossing"] ("External Ref Trigger")
              w241 = u8 0 items=["Fixed", "Linear", "Log"] ("SineOut Mode")
              w247 = u16 0 items=["Internal", "External"] ("Trigger Source (0: Internal)")
              w233 = u8 1 items=["Channel A", "Channel B"] ("OE1022D A/B")
              n67 = call "OE1022D_Configure Trigger.vi"("Trigger Source (0: Internal)"=w247, "error in (no error)   2"=w246, "OE1022D A/B"=w233, "VISA resource name   2"=w244) -> ("error out   2"=w259:errorcluster, "VISA resource name out   2"=w260:refnum<visa-resource-name>)
              n68 = call "OE1022D_Configure Reference Source.vi"("VISA resource name"=w260, "OE1022D A/B"=w233, "error in (no error)"=w259) -> ("VISA resource name out"=w258:refnum<visa-resource-name>, "error out"=w256:errorcluster)  [unwired: 15 in]
              n69 = call "OE1022D_Configure Harmonic.vi"("VISA resource name"=w258, "OE1022D A/B"=w233, "Harmonic 1"="1B harmonic 1", "Harmonic 2"="B harmonic 2", "error in (no error)"=w256) -> ("VISA resource name out"=w257:refnum<visa-resource-name>, "error out"=w255:errorcluster)  [unwired: 13 in]
              n70 = call "OE1022D_Configure Sine Out.vi"("VISA resource name"=w257, "SineOut Mode"=w241, "OE1022D A/B"=w233, "Sine Output Amplitude (V)"=sgl 0.0, "error in (no error)"=w255) -> ("VISA resource name out"=w262:refnum<visa-resource-name>, "error out"=w261:errorcluster)  [unwired: 9 in]
              n71 = call "OE1022D_Configure Frequency.vi"("VISA resource name"=w262, "OE1022D A/B"=w233, "Internal Frequency(Hz)"="1B frequency", "error in (no error)"=w261) -> ("VISA resource name out"=w254:refnum<visa-resource-name>, "error out"=w251:errorcluster)  [unwired: 14 in]
              n72 = call "OE1022D_Configure Ref Phase Channel B.vi"("VISA resource name"=w254, "Reference Source"="1B Reference Source", "External Ref Trigger"=w228, "Internal Frequency(Hz)"="1B frequency", "Auto Phase (T: Enabled)"="auto phase 1B", "error in (no error)"=w251, "Manual Phase  (degree)"="1B reference Manual Phase") -> ("VISA resource name out"=w253:refnum<visa-resource-name>, "error out"=w252:errorcluster)  [unwired: 11 in]
              n73 = call "OE1022D_Configure_Acquisition.vi"("VISA resource name"=w253, "OE1022D A/B"=w233, "Sample time (s)"="1B Sample time (s)", "error in (no error)"=w252, "Sample Mode (Single/Loop)"=w226) -> ("VISA resource name out"=w234:refnum<visa-resource-name>, "error out"=w235:errorcluster)  [unwired: 3 in]
              n74 = call "OE1022D_Configure Sensitivity.vi"("VISA resource name"=w234, "OE1022D A/B"=w233, "Sensitivity"="1B Sensitivity", "error in (no error)"=w235) -> ("VISA resource name out"=w238:refnum<visa-resource-name>, "error out"=w237:errorcluster)  [unwired: 14 in]
              n75 = call "OE1022D_Configure Filter.vi"("Low Pass Filter Slope (1: 12dB/oct)"="1B Low Pass Filter Slope", "Time Constant (8: 100ms)"="1B Time Constant", "error in (no error)"=w237, "Enable Sync Filter (F: Disable)"="Enable Sync Filter 1B (open f<200Hz)", "OE1022D A/B"=w233, "VISA resource name"=w238) -> ("error out"=w236:errorcluster, "VISA resource name out"=w225:refnum<visa-resource-name>)  [unwired: 4 in]
              n76 = call "OE1022D_Configure Input Filter.vi"("VISA resource name"=w225, "Input Source"="1B Input Connection (0: Single-Ended)", "OE1022D A/B"=w233, "error in (no error)"=w236) -> ("error out"=w245:errorcluster)  [unwired: 10 in, 1 out]
            }
            frame #3 {
              n77 = local read "stabilization(S)"() -> (w264:dbl)
              n78 = Multiply(x=w264, y=1000) -> (x*y=w266:dbl)
              n79 = Wait (ms)(milliseconds to wait=w266) -> ()  [unwired: 1 out]
            }
          }
        }
        frame #1 {
          n80 = for {
            N: w269 -> [_]
            shift-right: [w292] -> _
            shift-left: _ -> [w291]
            shift-right: [w287] -> _
            shift-left: _ -> [w286]
            shift-right: [w285] -> _
            shift-left: _ -> [w284]
            shift-right: [w283] -> _
            shift-left: _ -> [w282]
            shift-right: [w279] -> _
            shift-left: _ -> [w278]
            shift-right: [w277] -> _
            shift-left: _ -> [w276]
            shift-right: [w275] -> _
            shift-left: _ -> [w274]
            shift-right: [w273] -> _
            shift-left: _ -> [w272]
            tunnel: w268 -> [w271]
            tunnel: w267 -> [w270]
            i -> [w289]
            n81 = local read "Sine High Value (0.001-5V)"() -> (w281:dbl)
            n82 = local read "Sine Low Value (0V)"() -> (w280:dbl)
            n83 = Subtract(x=w281, y=w280) -> (x-y=w297:dbl)
            n84 = Add(x=1, y=w289) -> (x+y=→"loop run":i32)
            n85 = Divide(x="GATE STEP(mv)", y=1000) -> (x/y=w296:dbl)
            n86 = Divide(x=w297, y=w296) -> (x/y=w295:dbl)
            n87 = Multiply(x=2, y=w295) -> (x*y=w294:dbl)
            n88 = Increment(x=w294) -> (x+1=w293:dbl)
            n89 = for {
              N: w293 -> [_]
              tunnel: w296 -> [w337]
              shift-right: [w324] -> w292
              shift-left: w291 -> [w340]
              tunnel: w295 -> [w335]
              tunnel: w280 -> [w338]
              tunnel: w281 -> [w336]
              shift-right: [w323] -> _
              shift-left: _ -> [w328]
              shift-right: [w327] -> w287
              shift-left: w286 -> [w326]
              shift-right: [w322] -> w285
              shift-left: w284 -> [w321]
              shift-right: [w320] -> w283
              shift-left: w282 -> [w319]
              shift-right: [w312] -> w279
              shift-left: w278 -> [w309]
              shift-right: [w311] -> _
              shift-left: _ -> [w310]
              shift-right: [w308] -> w277
              shift-left: w276 -> [w307]
              shift-right: [w306] -> w275
              shift-left: w274 -> [w305]
              shift-right: [w304] -> w273
              shift-left: w272 -> [w303]
              tunnel: w271 -> [w302]
              tunnel: w270 -> [w301]
              i -> [w334]
              n90 = Less Or Equal?(x=w334, y=w335) -> (x <= y?=w339:bool)
              n91 = case shown="True" w339 {
                tunnel: w338 -> [w365 w393]
                tunnel: w334 -> [w374 w392]
                tunnel: w337 -> [w373 w391]
                tunnel: [w371 w389] -> w331
                tunnel: w336 -> [w372 _]
                tunnel: w335 -> [w367 _]
                tunnel: w334 -> [w370 _]
                frame False {
                  n92 = Multiply(x=w367, y=2) -> (x*y=w366:dbl)
                  n93 = Less Or Equal?(x=w370, y=w366) -> (x <= y?=w368:bool)
                  n94 = case shown="True" w368 {
                    tunnel: w374 -> [w381 w388]
                    tunnel: w373 -> [w379 w386]
                    tunnel: w372 -> [_ w384]
                    tunnel: [w377 w383] -> w371
                    tunnel: w367 -> [_ w382]
                    tunnel: w366 -> [w376 _]
                    tunnel: w365 -> [w375 _]
                    frame False {
                      n95 = Subtract(x=w381, y=w376) -> (x-y=w380:dbl)
                      n96 = Multiply(x=w379, y=w380) -> (x*y=w378:dbl)
                      n97 = Add(x=w375, y=w378) -> (x+y=w377:dbl)
                    }
                    frame True {
                      n98 = Subtract(x=w388, y=w382) -> (x-y=w387:dbl)
                      n99 = Multiply(x=w386, y=w387) -> (x*y=w385:dbl)
                      n100 = Subtract(x=w384, y=w385) -> (x-y=w383:dbl)
                    }
                  }
                }
                frame True {
                  n101 = Multiply(x=w391, y=w392) -> (x*y=w390:dbl)
                  n102 = Add(x=w393, y=w390) -> (x+y=w389:dbl)
                }
              }
              n103 = Absolute Value(x=w331) -> (abs(x)=w330:dbl)
              n104 = stacked-sequence {
                tunnel: w330 -> [w399 _ w420]
                tunnel: w340 -> [_ _ w484]
                tunnel: [_ _ w483] -> w324
                tunnel: [_ _ w482] -> w333
                tunnel: [_ _ w420] -> w332
                tunnel: [_ _ w481] -> w323
                tunnel: w328 -> [_ _ w480]
                tunnel: [_ _ w479] -> w329
                tunnel: [_ _ w478] -> w327
                tunnel: w326 -> [_ _ w471]
                tunnel: [_ _ w477] -> w322
                tunnel: w321 -> [_ _ w472]
                tunnel: [_ _ w476] -> w320
                tunnel: w319 -> [_ _ w475]
                tunnel: [_ _ w474] -> w318
                tunnel: [_ _ w473] -> w317
                tunnel: [_ _ w419] -> w316
                tunnel: [_ _ w418] -> w315
                tunnel: [_ _ w417] -> w314
                tunnel: [_ _ w416] -> w313
                tunnel: [_ _ w415] -> w312
                tunnel: [_ _ w414] -> w311
                tunnel: w310 -> [_ _ w413]
                tunnel: w309 -> [_ _ w412]
                tunnel: [_ _ w411] -> w308
                tunnel: w307 -> [_ _ w410]
                tunnel: [_ _ w409] -> w306
                tunnel: w305 -> [_ _ w408]
                tunnel: [_ _ w407] -> w304
                tunnel: w303 -> [_ _ w406]
                frame #0 {
                  n105 = Format Into String(format string="SLVLD1,%.3f;", w399) -> (resulting string=w397:string)  [unwired: 2 in, 1 out]
                  n106 = Concatenate Strings(w397, "\r") -> (w395:string)
                  n107 = local read "Two Lock-in ?"() -> (w394:bool)
                  n108 = case shown="True" w394 {
                    tunnel: w395 -> [_ w402]
                    frame False {
                    }
                    frame True {
                      n109 = local read "LOCKIN2 address"() -> (w401:refnum<visa-resource-name>)
                      n110 = VISA Write(VISA resource name=w401, write buffer=w402) -> ()  [unwired: 1 in, 3 out]
                    }
                  }
                  n111 = local read "LOCKIN1 address"() -> (w396:refnum<visa-resource-name>)
                  n112 = VISA Write(VISA resource name=w396, write buffer=w395) -> ()  [unwired: 1 in, 3 out]
                  "Sine voltage" <- w399
                }
                frame #1 {
                  n113 = Multiply(x="lockin waiting (s)", y=1000) -> (x*y=w405:dbl)
                  n114 = Wait (ms)(milliseconds to wait=w405) -> ()  [unwired: 1 out]
                }
                frame #2 {
                  n115 = local read "Two Lock-in ?"() -> (w421:bool)
                  n116 = case shown="True" w421 {
                    tunnel: w420 -> [_ w505]
                    tunnel: [w485 w504] -> w419
                    tunnel: [w485 w503] -> w418
                    tunnel: [w485 w502] -> w417
                    tunnel: [w485 w501] -> w416
                    tunnel: [w488 w500] -> w415
                    tunnel: [w490 w499] -> w414
                    tunnel: w413 -> [w490 w498]
                    tunnel: w412 -> [w488 w495]
                    tunnel: [w489 w497] -> w411
                    tunnel: w410 -> [w489 w496]
                    tunnel: [w487 w494] -> w409
                    tunnel: w408 -> [w487 w493]
                    tunnel: [w486 w492] -> w407
                    tunnel: w406 -> [w486 w491]
                    frame False {
                      w485 = nan
                    }
                    frame True {
                      n117 = flat-sequence {
                        tunnel: w505 -> [w582]
                        tunnel: w498 -> [w581]
                        tunnel: [w579] -> w554
                        tunnel: [w572] -> w553
                        tunnel: [w573] -> w552
                        tunnel: [w570] -> w551
                        tunnel: [w573] -> w550
                        tunnel: [w573] -> w549
                        tunnel: [w573] -> w548
                        tunnel: [w573] -> w547
                        tunnel: [w572] -> w546
                        tunnel: [w571] -> w545
                        tunnel: [w570] -> w544
                        tunnel: [w569] -> w543
                        tunnel: ["Clear Plot 2B"] -> w542
                        tunnel: ["Clear Plot 2A"] -> w541
                        tunnel: [w560] -> w540
                        tunnel: [w562] -> w539
                        tunnel: [w561] -> w538
                        tunnel: [w566] -> w537
                        tunnel: [w565] -> w536
                        tunnel: w496 -> [w556]
                        tunnel: w493 -> [w555]
                        tunnel: w554 -> [w604]
                        tunnel: [w604] -> w535
                        tunnel: w553 -> [w603]
                        tunnel: [w603] -> w534
                        tunnel: w552 -> [w602]
                        tunnel: [w602] -> w533
                        tunnel: w551 -> [w601]
                        tunnel: [w601] -> w532
                        tunnel: w550 -> [w600]
                        tunnel: [w600] -> w531
                        tunnel: w549 -> [w599]
                        tunnel: [w599] -> w530
                        tunnel: w548 -> [w598]
                        tunnel: [w598] -> w529
                        tunnel: w547 -> [w597]
                        tunnel: [w597] -> w528
                        tunnel: w546 -> [w596]
                        tunnel: [w596] -> w527
                        tunnel: w545 -> [w595]
                        tunnel: [w595] -> w526
                        tunnel: w544 -> [w594]
                        tunnel: [w594] -> w525
                        tunnel: w543 -> [w593]
                        tunnel: [w593] -> w524
                        tunnel: w542 -> [w592]
                        tunnel: [w592] -> w523
                        tunnel: w541 -> [w591]
                        tunnel: [w591] -> w522
                        tunnel: w540 -> [w590]
                        tunnel: [w590] -> w521
                        tunnel: w539 -> [w589]
                        tunnel: [w589] -> w520
                        tunnel: w538 -> [w588]
                        tunnel: [w588] -> w519
                        tunnel: w537 -> [w587]
                        tunnel: [w587] -> w518
                        tunnel: w536 -> [w586]
                        tunnel: [w586] -> w517
                        tunnel: w535 -> [w609]
                        tunnel: w534 -> [w642]
                        tunnel: w533 -> [w641]
                        tunnel: w532 -> [w640]
                        tunnel: w531 -> [w639]
                        tunnel: w530 -> [w637]
                        tunnel: w529 -> [w635]
                        tunnel: w528 -> [w633]
                        tunnel: w527 -> [w630]
                        tunnel: w526 -> [w629]
                        tunnel: w525 -> [w626]
                        tunnel: w524 -> [w625]
                        tunnel: w523 -> [w623]
                        tunnel: w491 -> [w621]
                        tunnel: w522 -> [w620]
                        tunnel: w521 -> [w616]
                        tunnel: w520 -> [w615]
                        tunnel: w519 -> [w614]
                        tunnel: w518 -> [w611]
                        tunnel: w517 -> [w610]
                        tunnel: [w609] -> w516
                        tunnel: [w628] -> w515
                        tunnel: [w642] -> w514
                        tunnel: [w641] -> w513
                        tunnel: [w607] -> w512
                        tunnel: [w608] -> w511
                        tunnel: [w631] -> w510
                        tunnel: [w627] -> w509
                        tunnel: [w624] -> w508
                        tunnel: [w640] -> w507
                        tunnel: [w613] -> w506
                        tunnel: w495 -> [w605]
                        tunnel: [w645] -> w501
                        tunnel: [w646] -> w503
                        tunnel: [w647] -> w494
                        tunnel: [w648] -> w500
                        tunnel: [w649] -> w492
                        tunnel: [w650] -> _
                        tunnel: [w651] -> w502
                        tunnel: [w652] -> w499
                        tunnel: [w653] -> w497
                        tunnel: [w654] -> _
                        tunnel: w516 -> [w654]
                        tunnel: w515 -> [w653]
                        tunnel: w514 -> [w643]
                        tunnel: w513 -> [w652]
                        tunnel: w512 -> [w651]
                        tunnel: w511 -> [w650]
                        tunnel: w510 -> [w649]
                        tunnel: w509 -> [w648]
                        tunnel: w508 -> [w647]
                        tunnel: w507 -> [w646]
                        tunnel: w506 -> [w645]
                        tunnel: [w643] -> w504
                        frame #0 {
                          w562 = u8 1 items=["Channel A", "Channel B"] ("Channel A/B for Parameter1")
                          w565 = u8 0 items=["Channel A", "Channel B"] ("Channel A/B for Parameter1")
                          n118 = local read "LOCKIN2 address"() -> (w557:refnum<visa-resource-name>)
                          n119 = Format Into String(0) -> (error out=w580:errorcluster)  [unwired: 3 in, 1 out]
                          n120 = Format Into String(0) -> (error out=w563:errorcluster)  [unwired: 3 in, 1 out]
                          n121 = call "OE1022D_Read 1 parameter_mean.vi"("错误输入（无错误）"=w580, "Parameter"="Parameter 2A", "Channel (0: A)"=w565, "VISA resource name"=w557) -> ("error out"=w566:errorcluster, "Measurement"=w574:dbl, "VISA resource name out"=w579:refnum<visa-resource-name>)  [unwired: 5 in]
                          n122 = call "OE1022D_Read 1 parameter_mean.vi"("Parameter 2"="Parameter 2B", "错误输入（无错误）"=w563, "Channel (0: A)"=w562, "VISA resource name"=w557) -> ("error out"=w560:errorcluster, "Measurement"=w559:dbl, "VISA resource name out"=w561:refnum<visa-resource-name>)  [unwired: 5 in]
                          n123 = Multiply(x=w574, y=1000.0) -> (x*y=w572:dbl)
                          "para2A Measurement" <- w572
                          n124 = Multiply(x=w559, y=1000000.0) -> (x*y=w570:dbl)
                          "para2B Measurement" <- w570
                          n125 = Build Array(w572) -> (w583:dbl[])
                          n126 = Build Array(w570) -> (w576:dbl[])
                          n127 = Select(t=w583, s="Clear Plot 2A", f=w556) -> (s? t:f=w571:dbl[])
                          n128 = Select(t=w576, s="Clear Plot 2B", f=w555) -> (s? t:f=w569:dbl[])
                          n129 = Build Array (concatenate)(w582, w581) -> (w573:dbl[])
                        }
                        frame #1 {
                          n130 = Wait (ms)(milliseconds to wait=u32 50) -> ()  [unwired: 1 out]
                        }
                        frame #2 {
                          n131 = Build Array (concatenate)(w630, w629) -> (w628:dbl[])
                          n132 = Build Array (concatenate)(w626, w625) -> (w624:dbl[])
                          n133 = Bundle(w635, w628) -> (→"XY Graph 7":cluster{dbl[], dbl[]})  [unwired: 1 in]
                          n134 = Bundle(w637, w624) -> (→"XY Graph 5":cluster{dbl[], dbl[]})  [unwired: 1 in]
                          n135 = call "OE1022D_Read 1 parameter_mean.vi"("错误输入（无错误）"=w611, "Parameter"="Phase 2A", "Channel (0: A)"=w610, "VISA resource name"=w609) -> ("error out"=w608:errorcluster, "Measurement"=w607:dbl)  [unwired: 5 in, 1 out]
                          "phase 2A" <- w607
                          n136 = call "OE1022D_Read 1 parameter_mean.vi"("Parameter 2"="Phase 2B", "错误输入（无错误）"=w616, "Channel (0: A)"=w615, "VISA resource name"=w614) -> ("Measurement"=w613:dbl)  [unwired: 5 in, 2 out]
                          "phase 2B" <- w613
                          n137 = Build Array(w607) -> (w617:dbl[])
                          n138 = Build Array(w613) -> (w618:dbl[])
                          n139 = Select(t=w617, s=w620, f=w621) -> (s? t:f=w619:dbl[])
                          n140 = Select(t=w618, s=w623, f=w605) -> (s? t:f=w622:dbl[])
                          n141 = Build Array (concatenate)(w607, w619) -> (w631:dbl[])
                          n142 = Build Array (concatenate)(w613, w622) -> (w627:dbl[])
                          n143 = Bundle(w633, w631) -> (→"XY Graph 8":cluster{dbl[], dbl[]})  [unwired: 1 in]
                          n144 = Bundle(w639, w627) -> (→"XY Graph 6":cluster{dbl[], dbl[]})  [unwired: 1 in]
                        }
                        frame #3 {
                          n145 = Wait (ms)(milliseconds to wait=u32 50) -> ()  [unwired: 1 out]
                        }
                      }
                    }
                  }
                  n146 = flat-sequence {
                    tunnel: w484 -> [w682]
                    tunnel: w420 -> [w681]
                    tunnel: w480 -> [w680]
                    tunnel: w475 -> [w674]
                    tunnel: [w678] -> w470
                    tunnel: [w670] -> w468
                    tunnel: [w671] -> w466
                    tunnel: [w668] -> w464
                    tunnel: [w671] -> w462
                    tunnel: [w671] -> w460
                    tunnel: [w671] -> w458
                    tunnel: [w671] -> w456
                    tunnel: [w670] -> w454
                    tunnel: [w669] -> w452
                    tunnel: [w668] -> w450
                    tunnel: [w667] -> w448
                    tunnel: ["Clear Plot 1B"] -> w446
                    tunnel: ["Clear Plot 1A"] -> w444
                    tunnel: [w658] -> w442
                    tunnel: [w660] -> w440
                    tunnel: [w659] -> w438
                    tunnel: [w664] -> w436
                    tunnel: [w663] -> w434
                    tunnel: w470 -> [w704]
                    tunnel: [w704] -> w469
                    tunnel: w468 -> [w703]
                    tunnel: [w703] -> w467
                    tunnel: w466 -> [w702]
                    tunnel: [w702] -> w465
                    tunnel: w464 -> [w701]
                    tunnel: [w701] -> w463
                    tunnel: w462 -> [w700]
                    tunnel: [w700] -> w461
                    tunnel: w460 -> [w699]
                    tunnel: [w699] -> w459
                    tunnel: w458 -> [w698]
                    tunnel: [w698] -> w457
                    tunnel: w456 -> [w697]
                    tunnel: [w697] -> w455
                    tunnel: w454 -> [w696]
                    tunnel: [w696] -> w453
                    tunnel: w452 -> [w695]
                    tunnel: [w695] -> w451
                    tunnel: w450 -> [w694]
                    tunnel: [w694] -> w449
                    tunnel: w448 -> [w693]
                    tunnel: [w693] -> w447
                    tunnel: w446 -> [w692]
                    tunnel: [w692] -> w445
                    tunnel: w444 -> [w691]
                    tunnel: [w691] -> w443
                    tunnel: w442 -> [w690]
                    tunnel: [w690] -> w441
                    tunnel: w440 -> [w689]
                    tunnel: [w689] -> w439
                    tunnel: w438 -> [w688]
                    tunnel: [w688] -> w437
                    tunnel: w436 -> [w687]
                    tunnel: [w687] -> w435
                    tunnel: w434 -> [w686]
                    tunnel: [w686] -> w433
                    tunnel: w469 -> [w708]
                    tunnel: w467 -> [w742]
                    tunnel: w465 -> [w741]
                    tunnel: w463 -> [w740]
                    tunnel: w461 -> [w739]
                    tunnel: w459 -> [w737]
                    tunnel: w457 -> [w735]
                    tunnel: w455 -> [w733]
                    tunnel: w453 -> [w730]
                    tunnel: w451 -> [w729]
                    tunnel: w449 -> [w726]
                    tunnel: w447 -> [w725]
                    tunnel: w472 -> [w723]
                    tunnel: w445 -> [w722]
                    tunnel: w471 -> [w720]
                    tunnel: w443 -> [w719]
                    tunnel: w441 -> [w715]
                    tunnel: w439 -> [w714]
                    tunnel: w437 -> [w713]
                    tunnel: w435 -> [w710]
                    tunnel: w433 -> [w709]
                    tunnel: [w708] -> w432
                    tunnel: [w728] -> w431
                    tunnel: [w742] -> w430
                    tunnel: [w741] -> w429
                    tunnel: [w706] -> w428
                    tunnel: [w707] -> w427
                    tunnel: [w731] -> w426
                    tunnel: [w727] -> w425
                    tunnel: [w724] -> w424
                    tunnel: [w740] -> w423
                    tunnel: [w712] -> w422
                    tunnel: [w744] -> w473
                    tunnel: [w745] -> w474
                    tunnel: [w746] -> w476
                    tunnel: [w747] -> w477
                    tunnel: [w748] -> w478
                    tunnel: [w749] -> _
                    tunnel: [w750] -> w479
                    tunnel: [w751] -> w481
                    tunnel: [w752] -> w482
                    tunnel: [w753] -> w483
                    tunnel: [w754] -> _
                    tunnel: w432 -> [w754]
                    tunnel: w431 -> [w753]
                    tunnel: w430 -> [w752]
                    tunnel: w429 -> [w751]
                    tunnel: w428 -> [w750]
                    tunnel: w427 -> [w749]
                    tunnel: w426 -> [w748]
                    tunnel: w425 -> [w747]
                    tunnel: w424 -> [w746]
                    tunnel: w423 -> [w745]
                    tunnel: w422 -> [w744]
                    frame #0 {
                      w660 = u8 1 items=["Channel A", "Channel B"] ("Channel A/B for Parameter1")
                      w663 = u8 0 items=["Channel A", "Channel B"] ("Channel A/B for Parameter1")
                      n147 = local read "LOCKIN1 address"() -> (w655:refnum<visa-resource-name>)
                      n148 = Format Into String(0) -> (error out=w679:errorcluster)  [unwired: 3 in, 1 out]
                      n149 = Format Into String(0) -> (error out=w661:errorcluster)  [unwired: 3 in, 1 out]
                      n150 = call "OE1022D_Read 1 parameter_mean.vi"("错误输入（无错误）"=w679, "Parameter"="Parameter 1A", "Channel (0: A)"=w663, "VISA resource name"=w655) -> ("error out"=w664:errorcluster, "Measurement"=w672:dbl, "VISA resource name out"=w678:refnum<visa-resource-name>)  [unwired: 5 in]
                      n151 = call "OE1022D_Read 1 parameter_mean.vi"("Parameter 2"="Parameter 1B", "错误输入（无错误）"=w661, "Channel (0: A)"=w660, "VISA resource name"=w655) -> ("error out"=w658:errorcluster, "Measurement"=w657:dbl, "VISA resource name out"=w659:refnum<visa-resource-name>)  [unwired: 5 in]
                      n152 = Multiply(x=w672, y=1000.0) -> (x*y=w670:dbl)
                      "para1A Measurement" <- w670
                      n153 = Multiply(x=w657, y=1000000.0) -> (x*y=w668:dbl)
                      "para1B Measurement" <- w668
                      n154 = Build Array(w670) -> (w683:dbl[])
                      n155 = Build Array(w668) -> (w675:dbl[])
                      n156 = Select(t=w683, s="Clear Plot 1A", f=w682) -> (s? t:f=w669:dbl[])
                      n157 = Select(t=w675, s="Clear Plot 1B", f=w674) -> (s? t:f=w667:dbl[])
                      n158 = Build Array (concatenate)(w681, w680) -> (w671:dbl[])
                    }
                    frame #1 {
                      n159 = Wait (ms)(milliseconds to wait=u32 50) -> ()  [unwired: 1 out]
                    }
                    frame #2 {
                      n160 = Build Array (concatenate)(w730, w729) -> (w728:dbl[])
                      n161 = Build Array (concatenate)(w726, w725) -> (w724:dbl[])
                      n162 = Bundle(w735, w728) -> (→"XY Graph":cluster{dbl[], dbl[]})  [unwired: 1 in]
                      n163 = Bundle(w737, w724) -> (→"XY Graph 3":cluster{dbl[], dbl[]})  [unwired: 1 in]
                      n164 = call "OE1022D_Read 1 parameter_mean.vi"("错误输入（无错误）"=w710, "Parameter"="Phase 1A", "Channel (0: A)"=w709, "VISA resource name"=w708) -> ("error out"=w707:errorcluster, "Measurement"=w706:dbl)  [unwired: 5 in, 1 out]
                      "phase 1A" <- w706
                      n165 = call "OE1022D_Read 1 parameter_mean.vi"("Parameter 2"="Phase 1B", "错误输入（无错误）"=w715, "Channel (0: A)"=w714, "VISA resource name"=w713) -> ("Measurement"=w712:dbl)  [unwired: 5 in, 2 out]
                      "phase 1B" <- w712
                      n166 = Build Array(w706) -> (w716:dbl[])
                      n167 = Build Array(w712) -> (w717:dbl[])
                      n168 = Select(t=w716, s=w719, f=w720) -> (s? t:f=w718:dbl[])
                      n169 = Select(t=w717, s=w722, f=w723) -> (s? t:f=w721:dbl[])
                      n170 = Build Array (concatenate)(w706, w718) -> (w731:dbl[])
                      n171 = Build Array (concatenate)(w712, w721) -> (w727:dbl[])
                      n172 = Bundle(w733, w731) -> (→"XY Graph 2":cluster{dbl[], dbl[]})  [unwired: 1 in]
                      n173 = Bundle(w739, w727) -> (→"XY Graph 4":cluster{dbl[], dbl[]})  [unwired: 1 in]
                    }
                    frame #3 {
                      n174 = Wait (ms)(milliseconds to wait=u32 50) -> ()  [unwired: 1 out]
                    }
                  }
                }
              }
              n175 = case shown="True" "Save data or not" {
                tunnel: w333 -> [_ w351]
                tunnel: w332 -> [_ w346]
                tunnel: w302 -> [_ w354]
                tunnel: w329 -> [_ w350]
                tunnel: w318 -> [_ w349]
                tunnel: w317 -> [_ w348]
                tunnel: w316 -> [_ w345]
                tunnel: w315 -> [_ w344]
                tunnel: w314 -> [_ w343]
                tunnel: w313 -> [_ w342]
                tunnel: w301 -> [_ w341]
                frame False {
                }
                frame True {
                  n176 = local read "Two Lock-in ?"() -> (w347:bool)
                  n177 = Build Array(w346, w351, w350, w349, w348) -> (w353:dbl[])
                  n178 = case shown="True" w347 {
                    tunnel: w346 -> [_ w361]
                    tunnel: w345 -> [_ w360]
                    tunnel: w344 -> [_ w359]
                    tunnel: w343 -> [_ w358]
                    tunnel: w342 -> [_ w357]
                    tunnel: w341 -> [_ w356]
                    frame False {
                    }
                    frame True {
                      n179 = Build Array(w361, w360, w358, w359, w357) -> (w363:dbl[])
                      n180 = call-poly <vilib>:"Write Delimited Spreadsheet.vi"("file path (dialog if empty)"=w356, "format (%.3f)"="%.10f", "1D data"=w363, "append to file? (new file:F)"=TRUE) -> ()  [unwired: 10 in, 2 out]
                    }
                  }
                  n181 = call-poly <vilib>:"Write Delimited Spreadsheet.vi"("file path (dialog if empty)"=w354, "format (%.3f)"="%.10f", "1D data"=w353, "append to file? (new file:F)"=TRUE) -> ()  [unwired: 10 in, 2 out]
                }
              }
            }
          }
        }
      }
    }
  }
  n182 = local read "Temperature \n& Field Function"() -> (w12:bool)
  n183 = local read "1A frequency"() -> (w14:dbl)
  n184 = Format Into String(format string="%.1f", w14) -> (resulting string=w5:string)  [unwired: 2 in, 1 out]
  n185 = case shown="False" w12 {
    tunnel: ["" w758] -> w4
    tunnel: ["" w757] -> w3
    frame False {
    }
    frame True {
      n186 = local read "Set  T  (K)"() -> (w761:dbl)
      n187 = Format Into String(format string="%.1f", w761) -> (resulting string=w758:string)  [unwired: 2 in, 1 out]
      n188 = local read "Set F (Oe)"() -> (w759:dbl)
      n189 = Format Into String(format string="%.1f", w759) -> (resulting string=w757:string)  [unwired: 2 in, 1 out]
    }
  }
  n190 = Format Into String(initial string="path1 (folder + filename)", "Series Resistance", w4, "K", w3, "Oe", w5, "Hz", ".txt") -> (resulting string=w17:string)  [unwired: 2 in, 1 out]
  n191 = String To Path(string=w17) -> (path=w16:path)
  n192 = Format Into String(initial string="path2 (folder + filename)", "Series Resistance", w4, "K", w3, "Oe", w5, "Hz", ".txt") -> (resulting string=w2:string)  [unwired: 2 in, 1 out]
  n193 = String To Path(string=w2) -> (path=w1:path)
